vi "Pose2DDistance.vi"(9 "Second Pose2D":T1, 11 "First Pose2D":T1) -> (2 "Distance":dbl)   [LabVIEW 2018]
uses:
  Pose2D.ctl
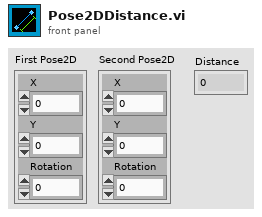
[diagram p1: front panel]
types:
  T1 = typedef "Pose2D.ctl" = cluster{"X":dbl, "Y":dbl, "Rotation":dbl}
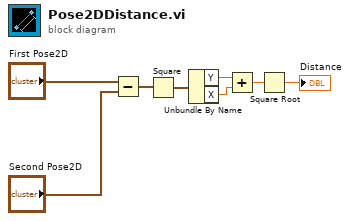
[diagram p0: block diagram]
diagram:
  n1 = Subtract(x="First Pose2D", y="Second Pose2D") -> (x-y=w1:T1)
  n2 = Square(x=w1) -> (x^2=w6:T1)
  n3 = Unbundle By Name(w6) -> ("Y"=w5:dbl, "X"=w4:dbl)
  n4 = Add(x=w5, y=w4) -> (x+y=w7:dbl)
  n5 = Square Root(x=w7) -> (sqrt(x)=→"Distance":dbl)
